vi "Long Execution Method.vi"(8 "error in (no error)":errorcluster, 11 "Async Actor Example in":refnum<class "Async Methods Actor Example.lvclass">) -> (0 "error out":errorcluster, 3 "Async Actor Example out":refnum<class "Async Methods Actor Example.lvclass">)   [LabVIEW 2021, in "Async Methods Actor Example.lvlib" / "Async Methods Actor Example.lvclass"]
uses:
  Async Methods Actor Example.lvclass
  Async Methods Actor Example.lvclass/Async Methods Actor Example.ctl
panel:
  in  "Stop":bool
  out "String":string
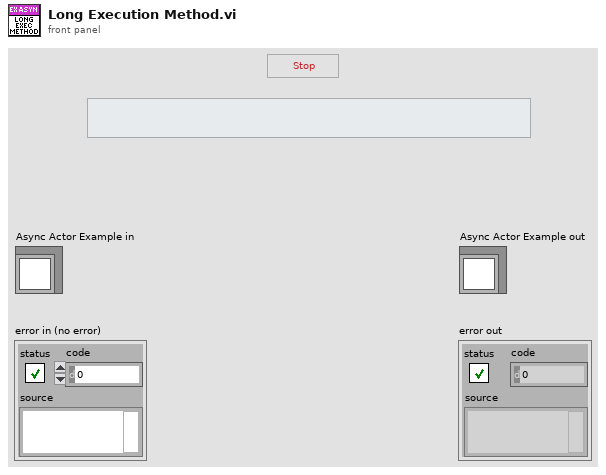
[diagram p1: front panel]
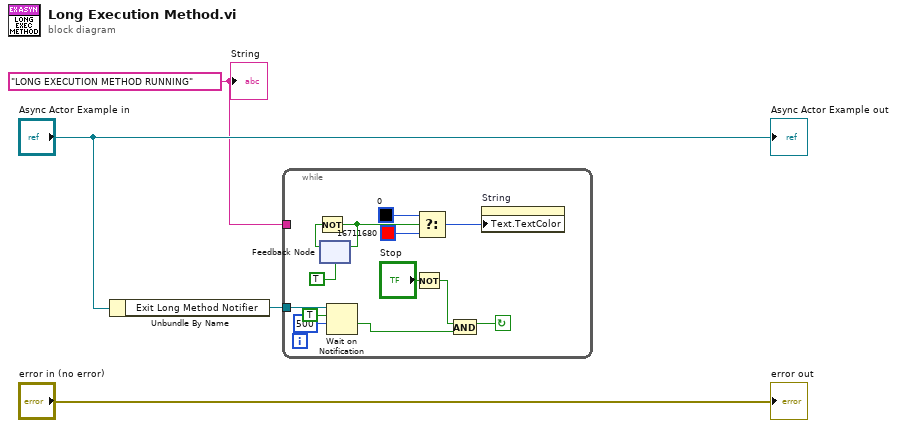
[diagram p0: block diagram]
diagram:
  w1 = "LONG EXECUTION METHOD RUNNING" ("String")
  n1 = Unbundle By Name("Async Actor Example in") -> ("Exit Long Method Notifier"=w2:refnum<notifier>)
  n2 = while {
    tunnel: w2 -> [w11]
    tunnel: w1 -> [_]
    stop <- w9 continue-if-true
    n3 = feedback #1(TRUE) -> (w16:bool)
    n4 = Not(x=w16) -> (.not. x?=w15:bool)
    n5 = feedback-in #1(w15) -> ()
    n6 = Wait on Notification(notifier=w11, ignore previous (F)=TRUE, timeout in ms (-1)=500) -> (timed out?=w8:bool)  [unwired: 1 in, 3 out]
    n7 = Not(x="Stop") -> (.not. x?=w6:bool)
    n8 = Select(t=u32 0 ("Text.Text Colors:Text Color"), s=w15, f=u32 16711680 ("Text.Text Colors:Text Color")) -> (s? t:f=w12:u32)
    n9 = And(x=w6, y=w8) -> (x .and. y?=w9:bool)
    n10 = property on="String" class="Str"("Text.TextColor"=w12) -> ()  [unwired: 2 in, 2 out]
  }
  "error out" <- "error in (no error)"
  "Async Actor Example out" <- "Async Actor Example in"
  "String" <- w1
